vi "Get Numerical Type.vi"() -> (3 "VI Numerical Type":string)   [LabVIEW 2012, in "OpenCLV x64.lvlib"]
uses:
  OpenCLV x64.lvlib
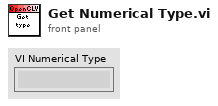
[diagram p1: front panel]
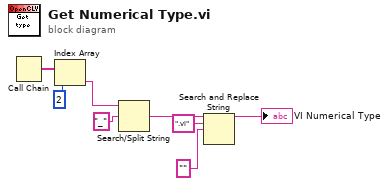
[diagram p0: block diagram]
diagram:
  n1 = Call Chain() -> (call chain=w7:string[])
  n2 = Index Array(array=w7, index=2) -> (element=w5:string)
  n3 = Search/Split String(string=w5, search string/char (-)="_" ("search string")) -> (match + rest of string=w4:string)  [unwired: 1 in, 2 out]
  n4 = Search and Replace String(input string=w4, search string=".vi", replace string="" ("replace string (\"\")")) -> (result string=→"VI Numerical Type":string)  [unwired: 5 in, 3 out]
